vi "DHE_DRV_fast_expose.vi"(0 "fd":i32, 9 "expt_time":u32, 11 "error in (no error)":errorcluster, 12 "frames_per_image":i32, 13 "nimages":i32) -> (4 "fd out":i32, 10 "return value":i32, 15 "error out":errorcluster)   [LabVIEW 2016]
doc: "This VI closes the I/O interface with the instrument."
uses:
  c/lib/libarcDHE.so
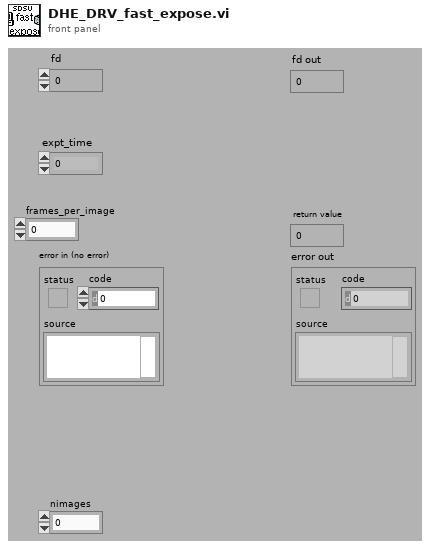
[diagram p1: front panel]
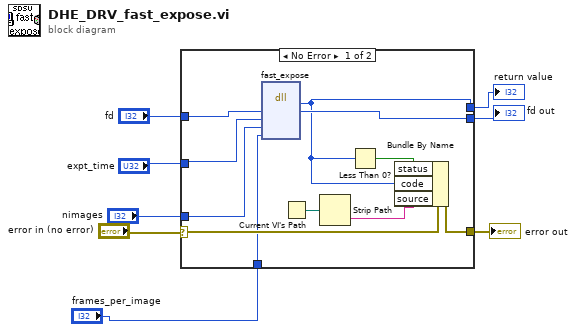
[diagram p0: block diagram]
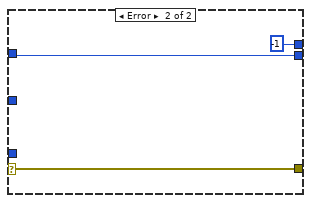
[diagram p2: hidden frame]
diagram:
  n1 = case shown="No Error" "error in (no error)" {
    selector: "error in (no error)" -> [w15 w21]
    tunnel: [w12 -1] -> w8
    tunnel: [w16 w21] -> w7
    tunnel: "fd" -> [w14 w20]
    tunnel: "expt_time" -> [w11 _]
    tunnel: [w13 w20] -> w3
    tunnel: "nimages" -> [w10 _]
    tunnel: "frames_per_image" -> [w9 _]
    frame No Error {
      n2 = dll-call lib="home/simager/panview/PAN/Modules/SDSU/private/c/lib/libarcDHE.so" fn="fast_expose"("fd"=w14, "exp_time"=w11, "nimages"=w10, "nir"=w9) -> ("return type"=w12:i32, "fd"=w13:i32)  [unwired: 6 in, 2 out]
      n3 = Current VI's Path() -> (path=w18:path)
      n4 = Strip Path(path=w18) -> (name=w17:string)  [unwired: 1 out]
      n5 = Less Than 0?(x=w12) -> (x < 0?=w19:bool)
      n6 = Bundle By Name(cluster=w15, "status"=w19, "code"=w12, "source"=w17) -> (w16:errorcluster)
    }
    frame Error {
    }
  }
  "error out" <- w7
  "return value" <- w8
  "fd out" <- w3
